vi "Mem1024_Fast2.vi"(6 "Reset":bool, 8 "Init":bool, 9 "Phi2":bool, 10 "Phi1":bool, 11 "In":bool) -> (0 "HexMap":u32[][](array[numeric]) format="%08b", 3 "Out":bool)   [LabVIEW 2012]
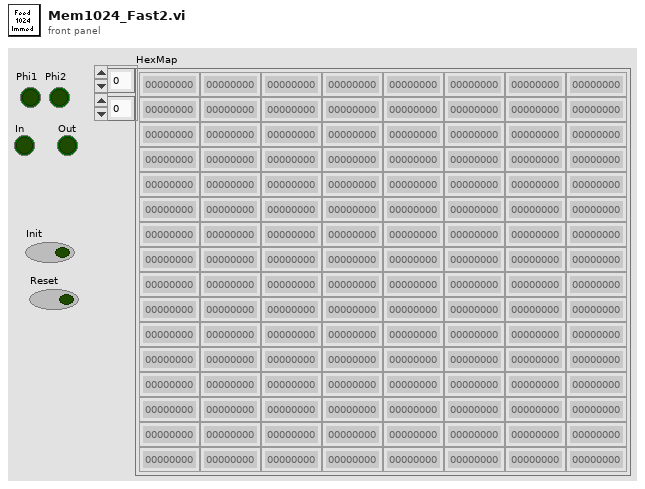
[diagram p1: front panel]
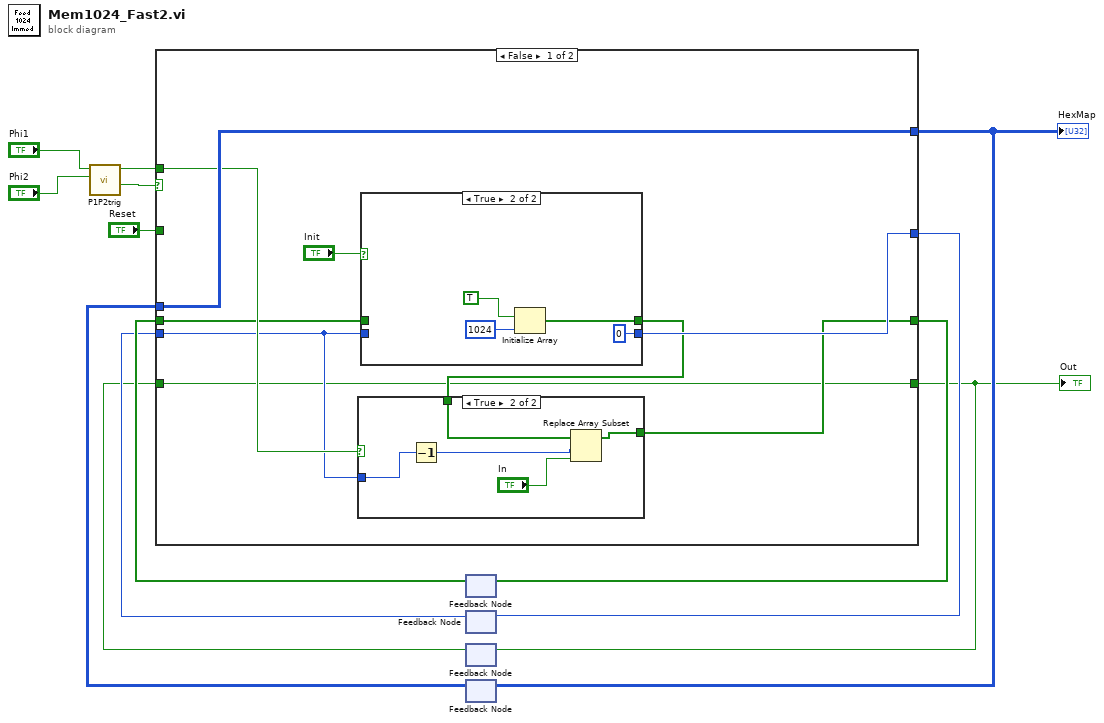
[diagram p0: block diagram]
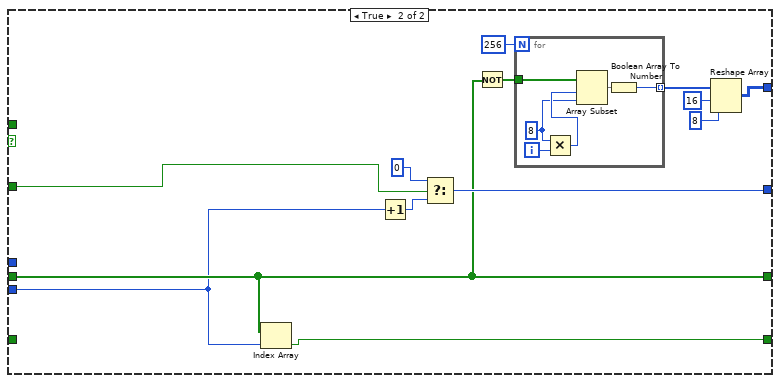
[diagram p4: hidden frame]
diagram:
  n1 = call "P1P2trig.vi"("Phi2"="Phi2", "Phi1"="Phi1") -> ("TrigUp"=w11:bool, "TrigDown"=w1:bool)  [unwired: 7 in, 1 out]
  n2 = feedback #1() -> (w10:bool[])  [unwired: 1 in]
  n3 = feedback #2() -> (w8:i32)  [unwired: 1 in]
  n4 = feedback #3() -> (w6:bool)  [unwired: 1 in]
  n5 = feedback #4() -> (w4:u32[][])  [unwired: 1 in]
  n6 = case shown="False" w11 {
    tunnel: w10 -> [w18 w36]
    tunnel: [w15 w36] -> w9
    tunnel: [w14 w37] -> w2
    tunnel: w8 -> [w17 w35]
    tunnel: [w21 w45] -> w7
    tunnel: w6 -> [w14 _]
    tunnel: [w20 w42] -> w5
    tunnel: w4 -> [w20 _]
    tunnel: "Reset" -> [_ w38]
    tunnel: w1 -> [w19 _]
    frame False {
      n7 = case shown="True" "Init" {
        tunnel: [w30 w32] -> w16
        tunnel: w18 -> [w30 _]
        tunnel: w17 -> [w29 _]
        tunnel: [w29 0 ("y")] -> w21
        frame False {
        }
        frame True {
          n8 = Initialize Array(TRUE, 1024 ("dimension size")) -> (w32:bool[])
        }
      }
      n9 = case shown="True" w19 {
        tunnel: [w23 w26] -> w15
        tunnel: w16 -> [w23 w25]
        tunnel: w17 -> [_ w28]
        frame False {
        }
        frame True {
          n10 = Decrement(x=w28) -> (x-1=w24:i32)
          n11 = Replace Array Subset(array=w25, new element="In", index=w24) -> (w26:bool[])
        }
      }
    }
    frame True {
      n12 = Index Array(array=w36, index=w35) -> (element=w37:bool)
      n13 = Increment(x=w35) -> (x+1=w46:i32)
      n14 = Select(t=0 ("y"), s=w38, f=w46) -> (s? t:f=w45:i32)
      n15 = Not(x=w36) -> (.not. x?=w39:bool[])
      n16 = for {
        N: 256 -> [_]
        tunnel: w39 -> [w53]
        tunnel: [w48] -> w43 mode=indexing
        i -> [w52]
        w50 = 8 ("x")
        n17 = Multiply(x=w50, y=w52) -> (x*y=w51:i32)
        n18 = Array Subset(array=w53, index=w51, length=w50) -> (w49:bool[])
        n19 = Boolean Array To Number(Boolean array=w49) -> (number=w48:u32)
      }
      n20 = Reshape Array(w43, 16 ("dimension size"), 8 ("dimension size")) -> (w42:u32[][])
    }
  }
  "Out" <- w2
  "HexMap" <- w5
  n21 = feedback-in #1(w9) -> ()
  n22 = feedback-in #2(w7) -> ()
  n23 = feedback-in #3(w2) -> ()
  n24 = feedback-in #4(w5) -> ()
